vi "ReportPart.vi"(6 "试验项目":enum32{"拉轴", "卡簧"}(ring), 8 "error in":errorcluster, 9 "索引IN":i32, 10 "合格":T1, 11 "report in":refnum<class "NI_report.lvclass">) -> (0 "error out 2":errorcluster caption="error out", 2 "索引OUT":i32, 3 "report out":refnum<class "NI_report.lvclass">)   [LabVIEW 2020]
uses:
  <vilib>/Utility/NIReport.llb/NI_report.lvclass
  OK.ctl
  <vilib>/Utility/NIReport.llb/image depth.ctl
  <vilib>/addons/_office/_exclsub.llb/font.ctl
  Global_Variable/Global.vi
  Global_Variable/A180648.vi
  <vilib>/Utility/NIReport.llb/Append Report Text (str wrap).vi
  <vilib>/addons/_office/word.llb/Word Easy Table (str).vi
  <vilib>/Utility/NIReport.llb/NI_ReportGenerationCore.lvlib
  <vilib>/addons/_office/NI_ReportGenerationToolkit.lvlib
  <vilib>/Utility/NIReport.llb/Word/NI_Word.lvclass
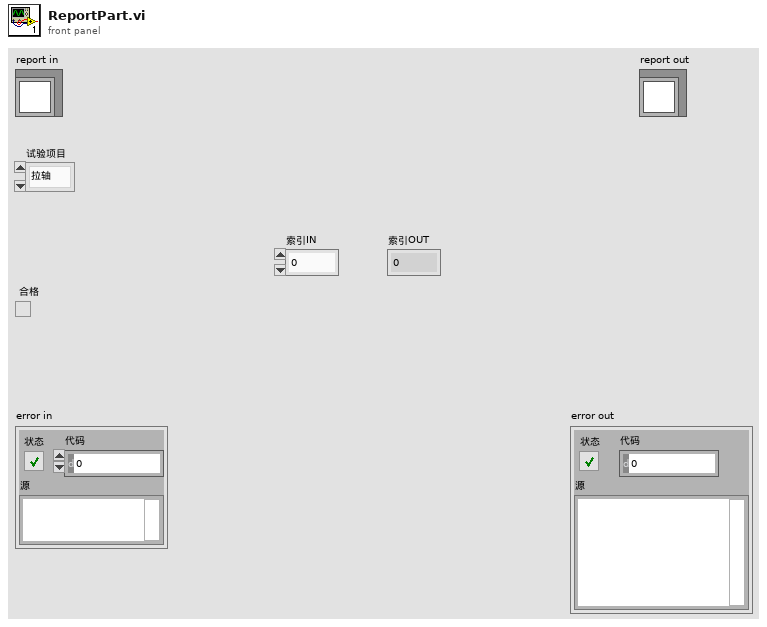
[diagram p1: front panel]
types:
  T1 = typedef "OK.ctl" = bool
  T2 = cluster{"Charset (-1)":i16, "Weight (-1)":i16, "Name":string, "Size":string}
  T3 = typedef "NI_ReportGenerationToolkit.lvlib/font.ctl" = cluster{"font name":string, "font size":dbl, "bold":u16, "italic":u16, "underline":u16, "strike through":u16, "font color":u32}
  T4 = cluster{"Italic":enum16{"Italic Unchanged", "Italic On", "Italic Off"}, "Strike Through":enum16{"Strike Through Unchanged", "Strike Through On", "Strike Through Off"}, "Underline":enum16{"Underline Unchanged", "Underline On", "Underline Off"}, "Bold":enum16{"Bold Unchanged", "Bold On", "Bold Off"}}
  T5 = typedef "NI_ReportGenerationCore.lvlib/image depth.ctl" = u16
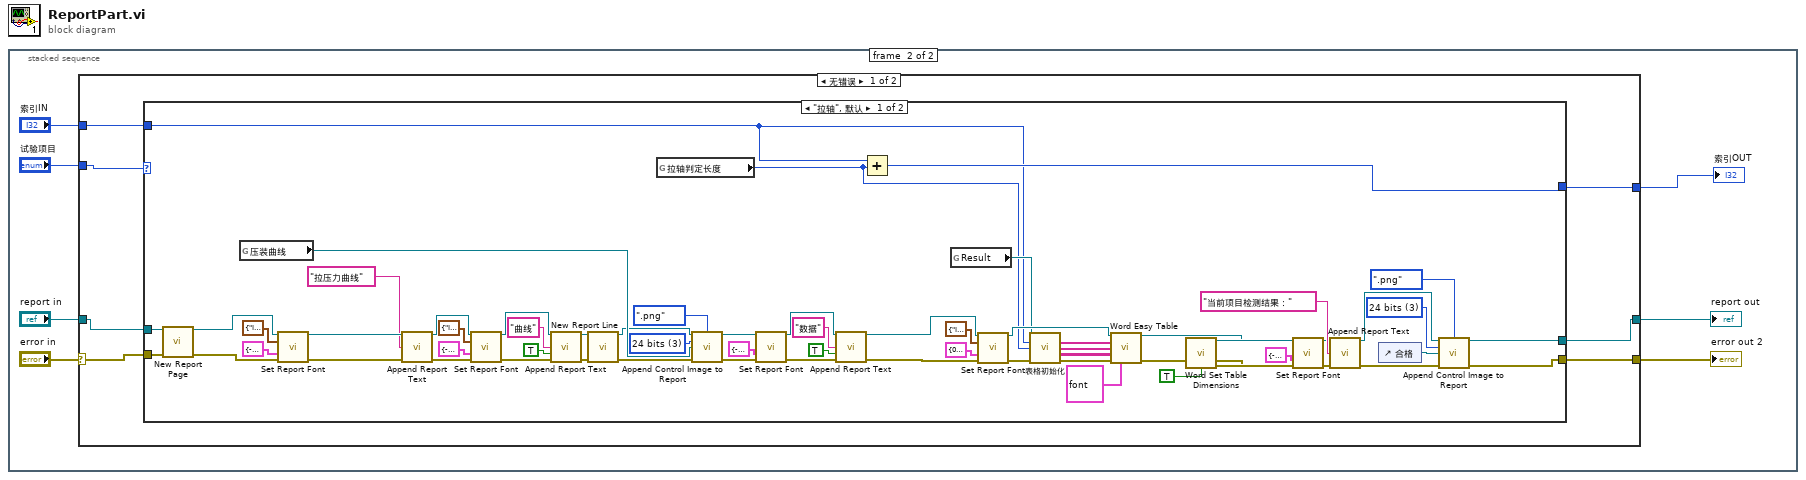
[diagram p0: block diagram]
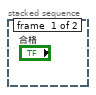
[diagram p2: hidden frame]
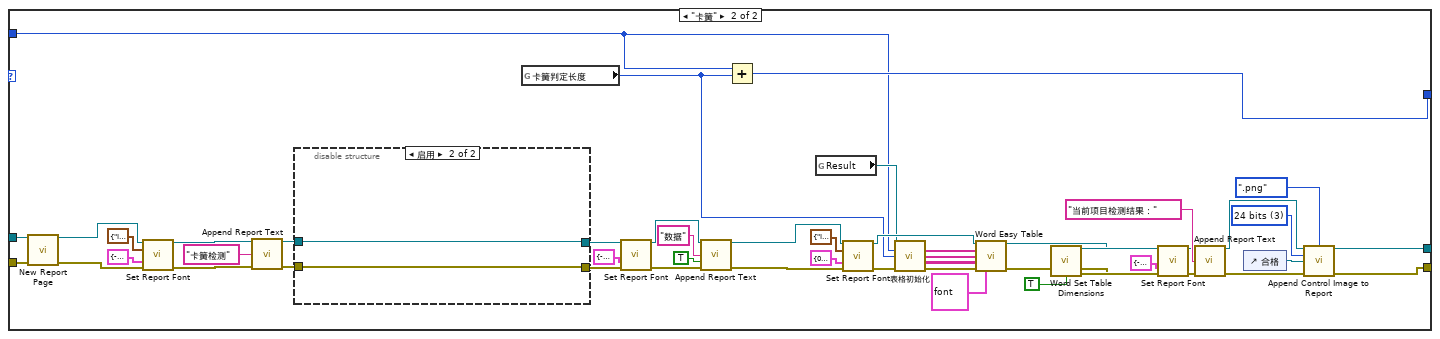
[diagram p3: hidden frame]
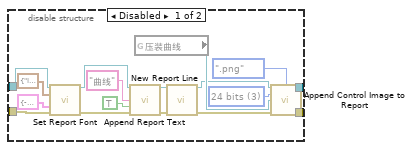
[diagram p4: hidden frame]
diagram:
  n1 = stacked-sequence {
    frame #0 {
    }
    frame #1 {
      n2 = case shown="无错误" "error in" {
        selector: "error in" -> [w14 w147]
        tunnel: [w13 w147] -> w6
        tunnel: "索引IN" -> [w9 w145]
        tunnel: "试验项目" -> [w8 _]
        tunnel: [w10 w145] -> w1
        tunnel: [w12 w146] -> w3
        tunnel: "report in" -> [w11 w146]
        frame No Error {
          n3 = case shown="\"拉轴\", 默认" w8 {
            tunnel: w14 -> [w69 w121]
            tunnel: [w64 w116] -> w13
            tunnel: [w39 w104] -> w12
            tunnel: w11 -> [w38 w103]
            tunnel: [w36 w101] -> w10
            tunnel: w9 -> [w16 w81]
            frame "拉轴", Default {
              w52 = T5 3 items=["B&W", "4 bits", "8 bits", "24 bits"] ("image depth")
              w62 = T5 3 items=["B&W", "4 bits", "8 bits", "24 bits"] ("image depth")
              n4 = call-dynamic "New Report Page.vi"("report in"=w38, "error in (no error)"=w69) -> ("report out"=w67:refnum<class "NI_report.lvclass">, "error out"=w68:errorcluster)  [unwired: 12 in]
              n5 = global read "A180648.vi" "压装曲线"() -> (w55:refnum<vi>)
              n6 = call-dynamic "Set Report Font.vi"("report in"=w67, "text options"=T4 {"Italic"=enum."Italic Unchanged", "Strike Through"=enum."Strike Through Unchanged", "Underline"=enum."Underline Unchanged", "Bold"=enum."Bold On"}, "font settings"=T2 {"Charset (-1)"=-1, "Weight (-1)"=-1, "Name"="楷体", "Size"="16 "}, "error in (no error)"=w68) -> ("report out"=w76:refnum<class "NI_report.lvclass">, "error out"=w75:errorcluster)  [unwired: 9 in, 1 out]
              n7 = call-poly <vilib>:"Append Report Text.vi"("report in"=w76, "text"="拉压力曲线", "error in (no error)"=w75) -> ("report out"=w71:refnum<class "NI_report.lvclass">, "error out"=w70:errorcluster)  [unwired: 9 in, 2 out]
              n8 = call-dynamic "Set Report Font.vi"("report in"=w71, "text options"=T4 {"Italic"=enum."Italic Unchanged", "Strike Through"=enum."Strike Through Unchanged", "Underline"=enum."Underline Unchanged", "Bold"=enum."Bold Off"}, "font settings"=T2 {"Charset (-1)"=-1, "Weight (-1)"=-1, "Name"="宋体", "Size"="12"}, "error in (no error)"=w70) -> ("report out"=w46:refnum<class "NI_report.lvclass">, "error out"=w43:errorcluster)  [unwired: 9 in, 1 out]
              n9 = call-poly <vilib>:"Append Report Text.vi"("report in"=w46, "text"="曲线", "append on new line? (F)"=TRUE, "error in (no error)"=w43) -> ("report out"=w45:refnum<class "NI_report.lvclass">, "error out"=w44:errorcluster)  [unwired: 8 in, 2 out]
              n10 = call-dynamic "New Report Line.vi"("report in"=w45, "error in (no error)"=w44) -> ("report out"=w53:refnum<class "NI_report.lvclass">, "error out"=w54:errorcluster)  [unwired: 12 in]
              n11 = global read "判定参数.vi" "拉轴判定长度"() -> (w15:i32)
              n12 = call-dynamic "Append Control Image to Report.vi"("report in"=w53, "image file type (.jpg)"=enum16{".jpg", ".png"}.".png", "image depth"=w52, "ctrl reference"=w55, "error in (no error)"=w54) -> ("report out"=w50:refnum<class "NI_report.lvclass">, "error out"=w49:errorcluster)  [unwired: 7 in, 2 out]
              n13 = call-dynamic "Set Report Font.vi"("report in"=w50, "font settings"=T2 {"Charset (-1)"=-1, "Weight (-1)"=-1, "Name"="微软雅黑", "Size"="12 "}, "error in (no error)"=w49) -> ("report out"=w35:refnum<class "NI_report.lvclass">, "error out"=w32:errorcluster)  [unwired: 10 in, 1 out]
              n14 = call-poly <vilib>:"Append Report Text.vi"("report in"=w35, "text"="数据", "append on new line? (F)"=TRUE, "error in (no error)"=w32) -> ("report out"=w18:refnum<class "NI_report.lvclass">, "error out"=w17:errorcluster)  [unwired: 8 in, 2 out]
              n15 = Add(x=w16, y=w15) -> (x+y=w36:i32)
              n16 = global read "Global.vi" "Result"() -> (w19:refnum<vi>)
              n17 = call-dynamic "Set Report Font.vi"("report in"=w18, "text options"=T4 {"Italic"=enum."Italic Unchanged", "Strike Through"=enum."Strike Through Unchanged", "Underline"=enum."Underline Unchanged", "Bold"=enum."Bold Unchanged"}, "font settings"=T2 {"Charset (-1)"=0, "Weight (-1)"=-1, "Name"="微软雅黑", "Size"="12 "}, "error in (no error)"=w17) -> ("report out"=w21:refnum<class "NI_report.lvclass">, "error out"=w20:errorcluster)  [unwired: 9 in, 1 out]
              n18 = call "表格初始化.vi"("表格引用"=w19, "索引"=w16, "长度"=w15, "错误输入（无错误）"=w20) -> ("行首字符串[]"=w23:string[], "列首字符串[]"=w22:string[], "文本数据"=w25:string[][], "错误输出"=w28:errorcluster)  [unwired: 7 in, 1 out]
              n19 = call-poly <vilib>:"Word Easy Table.vi"("report in"=w21, "row headers"=w23, "column headers"=w22, "data"=w25, "error in (no error)"=w28, "font"=T3 {"font name"="宋体", "font size"=12.0, "bold"=2, "italic"=2, "underline"=2, "strike through"=2, "font color"=16777216}) -> ("report out"=w26:refnum<class "NI_report.lvclass">, "error out"=w27:errorcluster)  [unwired: 7 in, 1 out]
              n20 = call <vilib>:"Word Set Table Dimensions.vi"("report in"=w26, "error in (no error)"=w27, "fit to page width? (F)"=TRUE) -> ("report out"=w57:refnum<class "NI_report.lvclass">, "error out"=w56:errorcluster)  [unwired: 11 in]
              n21 = call-dynamic "Set Report Font.vi"("report in"=w57, "font settings"=T2 {"Charset (-1)"=-1, "Weight (-1)"=-1, "Name"="宋体", "Size"="16 "}, "error in (no error)"=w56) -> ("report out"=w60:refnum<class "NI_report.lvclass">, "error out"=w61:errorcluster)  [unwired: 10 in, 1 out]
              n22 = call-poly <vilib>:"Append Report Text.vi"("report in"=w60, "text"="当前项目检测结果：", "error in (no error)"=w61) -> ("report out"=w66:refnum<class "NI_report.lvclass">, "error out"=w65:errorcluster)  [unwired: 9 in, 2 out]
              n23 = control-ref of="合格"() -> (w37:refnum<vi>)
              n24 = call-dynamic "Append Control Image to Report.vi"("report in"=w66, "image file type (.jpg)"=enum16{".jpg", ".png"}.".png", "image depth"=w62, "ctrl reference"=w37, "error in (no error)"=w65) -> ("report out"=w39:refnum<class "NI_report.lvclass">, "error out"=w64:errorcluster)  [unwired: 7 in, 2 out]
            }
            frame "卡簧" {
              w114 = T5 3 items=["B&W", "4 bits", "8 bits", "24 bits"] ("image depth")
              n25 = call-dynamic "New Report Page.vi"("report in"=w103, "error in (no error)"=w121) -> ("report out"=w119:refnum<class "NI_report.lvclass">, "error out"=w120:errorcluster)  [unwired: 12 in]
              n26 = call-dynamic "Set Report Font.vi"("report in"=w119, "text options"=T4 {"Italic"=enum."Italic Unchanged", "Strike Through"=enum."Strike Through Unchanged", "Underline"=enum."Underline Unchanged", "Bold"=enum."Bold On"}, "font settings"=T2 {"Charset (-1)"=-1, "Weight (-1)"=-1, "Name"="楷体", "Size"="16 "}, "error in (no error)"=w120) -> ("report out"=w125:refnum<class "NI_report.lvclass">, "error out"=w124:errorcluster)  [unwired: 9 in, 1 out]
              n27 = call-poly <vilib>:"Append Report Text.vi"("report in"=w125, "text"="卡簧检测", "error in (no error)"=w124) -> ("report out"=w79:refnum<class "NI_report.lvclass">, "error out"=w78:errorcluster)  [unwired: 9 in, 2 out]
              n28 = disable-structure shown="启用" {
                disable-tunnel: [w142 w144] -> w106
                disable-tunnel: [w141 w143] -> w105
                disable-tunnel: w79 -> [w140 w144]
                disable-tunnel: w78 -> [w139 w143]
                frame Disabled {
                  w135 = T5 3 items=["B&W", "4 bits", "8 bits", "24 bits"] ("image depth")
                  n29 = call-dynamic "Set Report Font.vi"("report in"=w140, "text options"=T4 {"Italic"=enum."Italic Unchanged", "Strike Through"=enum."Strike Through Unchanged", "Underline"=enum."Underline Unchanged", "Bold"=enum."Bold Off"}, "font settings"=T2 {"Charset (-1)"=-1, "Weight (-1)"=-1, "Name"="宋体", "Size"="12"}, "error in (no error)"=w139) -> ("report out"=w132:refnum<class "NI_report.lvclass">, "error out"=w129:errorcluster)  [unwired: 9 in, 1 out]
                  n30 = call-poly <vilib>:"Append Report Text.vi"("report in"=w132, "text"="曲线", "append on new line? (F)"=TRUE, "error in (no error)"=w129) -> ("report out"=w131:refnum<class "NI_report.lvclass">, "error out"=w130:errorcluster)  [unwired: 8 in, 2 out]
                  n31 = global read "A180648.vi" "压装曲线"() -> (w138:refnum<vi>)
                  n32 = call-dynamic "New Report Line.vi"("report in"=w131, "error in (no error)"=w130) -> ("report out"=w136:refnum<class "NI_report.lvclass">, "error out"=w137:errorcluster)  [unwired: 12 in]
                  n33 = call-dynamic "Append Control Image to Report.vi"("report in"=w136, "image file type (.jpg)"=enum16{".jpg", ".png"}.".png", "image depth"=w135, "ctrl reference"=w138, "error in (no error)"=w137) -> ("report out"=w142:refnum<class "NI_report.lvclass">, "error out"=w141:errorcluster)  [unwired: 7 in, 2 out]
                }
                frame Enabled {
                }
              }
              n34 = global read "判定参数.vi" "卡簧判定长度"() -> (w77:i32)
              n35 = call-dynamic "Set Report Font.vi"("report in"=w106, "font settings"=T2 {"Charset (-1)"=-1, "Weight (-1)"=-1, "Name"="微软雅黑", "Size"="12 "}, "error in (no error)"=w105) -> ("report out"=w100:refnum<class "NI_report.lvclass">, "error out"=w97:errorcluster)  [unwired: 10 in, 1 out]
              n36 = call-poly <vilib>:"Append Report Text.vi"("report in"=w100, "text"="数据", "append on new line? (F)"=TRUE, "error in (no error)"=w97) -> ("report out"=w83:refnum<class "NI_report.lvclass">, "error out"=w82:errorcluster)  [unwired: 8 in, 2 out]
              n37 = Add(x=w81, y=w77) -> (x+y=w101:i32)
              n38 = global read "Global.vi" "Result"() -> (w84:refnum<vi>)
              n39 = call-dynamic "Set Report Font.vi"("report in"=w83, "text options"=T4 {"Italic"=enum."Italic Unchanged", "Strike Through"=enum."Strike Through Unchanged", "Underline"=enum."Underline Unchanged", "Bold"=enum."Bold Unchanged"}, "font settings"=T2 {"Charset (-1)"=0, "Weight (-1)"=-1, "Name"="微软雅黑", "Size"="12 "}, "error in (no error)"=w82) -> ("report out"=w86:refnum<class "NI_report.lvclass">, "error out"=w85:errorcluster)  [unwired: 9 in, 1 out]
              n40 = call "表格初始化.vi"("表格引用"=w84, "索引"=w81, "长度"=w77, "错误输入（无错误）"=w85) -> ("行首字符串[]"=w88:string[], "列首字符串[]"=w87:string[], "文本数据"=w90:string[][], "错误输出"=w93:errorcluster)  [unwired: 7 in, 1 out]
              n41 = call-poly <vilib>:"Word Easy Table.vi"("report in"=w86, "row headers"=w88, "column headers"=w87, "data"=w90, "error in (no error)"=w93, "font"=T3 {"font name"="宋体", "font size"=12.0, "bold"=2, "italic"=2, "underline"=2, "strike through"=2, "font color"=16777216}) -> ("report out"=w91:refnum<class "NI_report.lvclass">, "error out"=w92:errorcluster)  [unwired: 7 in, 1 out]
              n42 = call <vilib>:"Word Set Table Dimensions.vi"("report in"=w91, "error in (no error)"=w92, "fit to page width? (F)"=TRUE) -> ("report out"=w109:refnum<class "NI_report.lvclass">, "error out"=w108:errorcluster)  [unwired: 11 in]
              n43 = call-dynamic "Set Report Font.vi"("report in"=w109, "font settings"=T2 {"Charset (-1)"=-1, "Weight (-1)"=-1, "Name"="宋体", "Size"="16 "}, "error in (no error)"=w108) -> ("report out"=w112:refnum<class "NI_report.lvclass">, "error out"=w113:errorcluster)  [unwired: 10 in, 1 out]
              n44 = call-poly <vilib>:"Append Report Text.vi"("report in"=w112, "text"="当前项目检测结果：", "error in (no error)"=w113) -> ("report out"=w118:refnum<class "NI_report.lvclass">, "error out"=w117:errorcluster)  [unwired: 9 in, 2 out]
              n45 = control-ref of="合格"() -> (w102:refnum<vi>)
              n46 = call-dynamic "Append Control Image to Report.vi"("report in"=w118, "image file type (.jpg)"=enum16{".jpg", ".png"}.".png", "image depth"=w114, "ctrl reference"=w102, "error in (no error)"=w117) -> ("report out"=w104:refnum<class "NI_report.lvclass">, "error out"=w116:errorcluster)  [unwired: 7 in, 2 out]
            }
          }
        }
        frame Error {
        }
      }
      "error out 2" <- w6
      "索引OUT" <- w1
      "report out" <- w3
    }
  }
